vi "Main.vi"(8 "error in (no error)":errorcluster, 11 "VISA resource name":refnum<visa-resource-name>) -> (0 "error out":errorcluster, 2 "Volume and Flow":string)   [LabVIEW 2016]
uses:
  <vilib>/Instr/_visa.llb/VISA Configure Serial Port (Instr).vi
panel:
  out "Type+Status":string
  in  "stop":bool
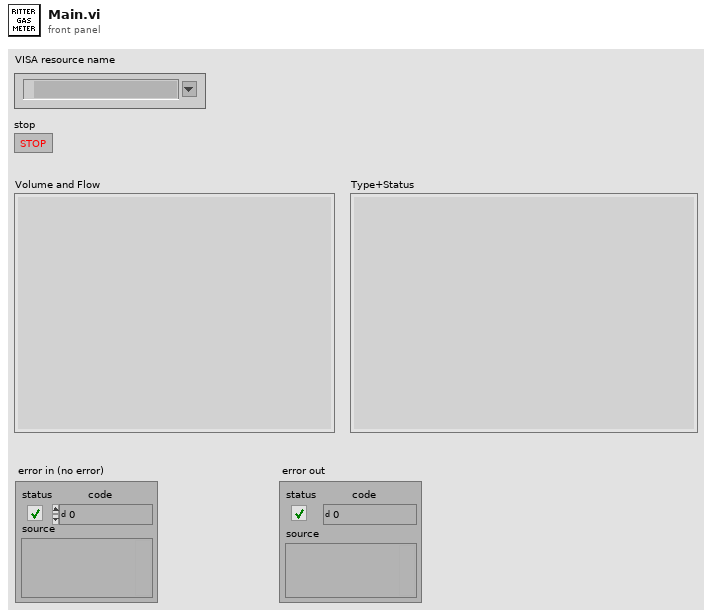
[diagram p1: front panel]
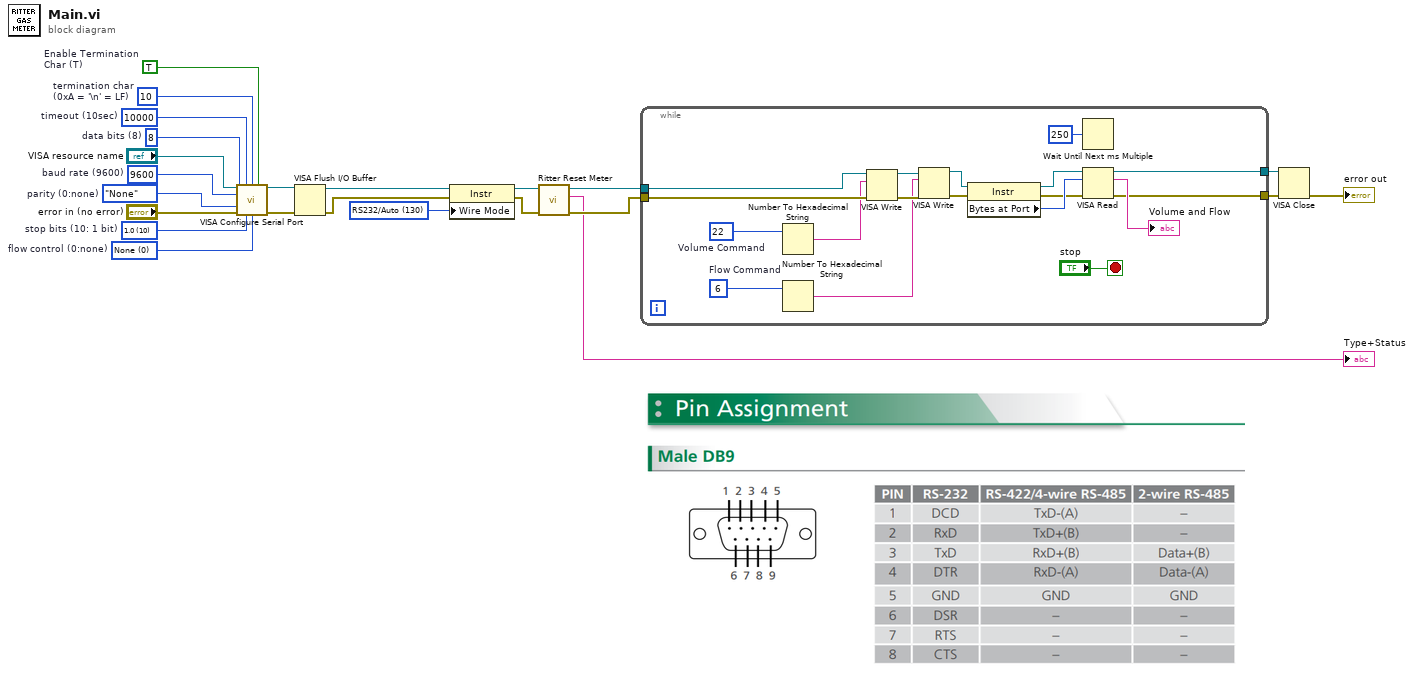
[diagram p0: block diagram]
diagram:
  w9 = TRUE  # Enable Termination Char (T)
  w10 = u8 10  # termination char (0xA = '\n' = LF)
  w11 = u32 10000  # timeout (10sec)
  w12 = u16 0 items=["None", "XON/XOFF", "RTS/CTS", "XON/XOFF & RTS/CTS", "DTR/DSR", "XON/XOFF & DTR/DSR"]  # flow control (0:none)
  w13 = u16 10 items=["1.0"=10, "1.5"=15, "2.0"=20]  # stop bits (10: 1 bit)
  w14 = enum16{"None", "Odd", "Even", "Mark", "Space"}."None"  # parity (0:none)
  w15 = u16 8  # data bits (8)
  w16 = u32 9600  # baud rate (9600)
  w23 = i16 130 items=["Unknown"=-1, "RS485/Wire4"=0, "RS485/Wire2-EchoDTR"=1, "RS485/Wire2-CtrlDTR"=2, "RS485/Wire2-Auto"=3, "RS232/DTE"=128, "RS232/DCE"=129, "RS232/Auto"=130] ("Serial Settings:Wire Mode")
  n1 = call-poly "VISA Configure Serial Port"("VISA resource name"="VISA resource name", "timeout (10sec)"=w11, "termination char\n(0xA = '\\n' = LF)"=w10, "Enable Termination\nChar (T)"=w9, "baud rate (9600)"=w16, "data bits (8)"=w15, "parity (0:none)"=w14, "error in (no error)"="error in (no error)", "stop bits (10: 1 bit)"=w13, "flow control (0:none)"=w12) -> ("VISA resource name out"=w20:refnum<visa-resource-name>, "error out"=w22:errorcluster)  [unwired: 4 in]
  n2 = VISA Flush I/O Buffer(VISA resource name=w20, error in (no error)=w22) -> (VISA resource name out=w19:refnum<visa-resource-name>, error out=w21:errorcluster)  [unwired: 1 in]
  n3 = property class="Instr"(reference=w19, error in=w21, "Wire Mode"=w23) -> (reference out=w5:refnum<visa-resource-name>, error out=w4:errorcluster)
  n4 = call "Ritter Reset Meter.vi"("error in (no error)"=w4, "VISA resource name"=w5) -> ("error out"=w2:errorcluster, "Type+Status"=→"Type+Status":string, "VISA resource name Output"=w3:refnum<visa-resource-name>)  [unwired: 7 in]
  n5 = while {
    tunnel: w3 -> [w30]
    tunnel: w2 -> [w31]
    tunnel: [w39] -> w17
    tunnel: [w35] -> w18
    stop <- "stop" stop-if-true
    w32 = u8 6  # Flow Command
    w33 = u8 22  # Volume Command
    n6 = Number To Hexadecimal String(2:w33) -> (0:w29:string)  [unwired: 1 in]
    n7 = Number To Hexadecimal String(2:w32) -> (0:w26:string)  [unwired: 1 in]
    n8 = VISA Write(VISA resource name=w30, write buffer=w29, error in (no error)=w31) -> (VISA resource name out=w27:refnum<visa-resource-name>, error out=w28:errorcluster)  [unwired: 1 out]
    n9 = VISA Write(VISA resource name=w27, write buffer=w26, error in (no error)=w28) -> (VISA resource name out=w24:refnum<visa-resource-name>, error out=w25:errorcluster)  [unwired: 1 out]
    n10 = property class="Instr"(reference=w24, error in=w25) -> (reference out=w41:refnum<visa-resource-name>, error out=w34:errorcluster, "Bytes at Port"=w40:u32)
    n11 = Wait Until Next ms Multiple(millisecond multiple=u32 250) -> ()  [unwired: 1 out]
    n12 = VISA Read(VISA resource name=w41, byte count=w40, error in (no error)=w34) -> (VISA resource name out=w39:refnum<visa-resource-name>, read buffer=→"Volume and Flow":string, error out=w35:errorcluster)  [unwired: 1 out]
  }
  n13 = VISA Close(VISA resource name=w17, error in (no error)=w18) -> (error out=→"error out":errorcluster)
